vi "Rename Error SMO Private Events.vi"(8 "error in (no error)":errorcluster, 10 "Public Events":T1) -> (0 "error out":errorcluster, 2 "Error SMO Public Events":T1)   [LabVIEW 2019, in "Instrument.lvclass"]
uses:
  Instrument.lvclass
  <vilib>/JKI/JKI SMO/SMO/Typedefs/Public Events.ctl
  <vilib>/JKI/JKI SMO/SMO/Typedefs/SMOState --Enum.ctl
  <vilib>/JKI/JKI SMO/SMO/Typedefs/Reserve State--Enum.ctl
  <vilib>/JKI/JKI SMO/SMO/SMO.lvclass
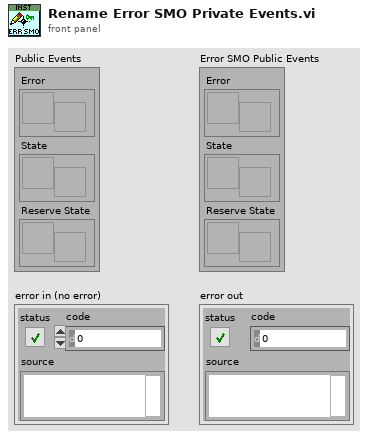
[diagram p1: front panel]
types:
  T1 = typedef "SMO.lvclass/Public Events.ctl" = cluster{"Error":refnum<user-event>, "State":refnum<user-event>, "Reserve State":refnum<user-event>}
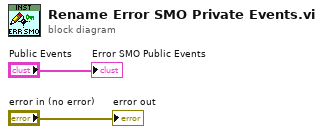
[diagram p0: block diagram]
diagram:
  "Error SMO Public Events" <- "Public Events"
  "error out" <- "error in (no error)"
